vi "Measurement_R2.vi"(0 "I offset":dbl, 1 "PID gains":T1={"proportional gain (Kc)"=1.0, "integral time (Ti, min)"=0.01, "derivative time (Td, min)"=0.0} {"derivative time (Td, min)" format="%.3f"; "integral time (Ti, min)" format="%.3f"; "proportional gain (Kc)" format="%.3f"}, 2 "input cluster":T2) -> (3 "VR frequency":dbl, 4 "VL frequency":dbl, 5 "PLL output":cluster{dbl, dbl, dbl, dbl}, 6 "RMS values":dbl[](array[numeric]), 8 "Total power values":dbl[](array[numeric]))   [LabVIEW 2016]
uses:
  <vilib>/ptbypt/NI_PtbyPt.lvlib
panel:
  out "RMS":fxp<+,55,5>
  in  "output cluster":cluster{"reinitialize? (F)":bool, "dt (s)":dbl}
  out "I RMS":dbl
  out "VR RMS":dbl
  out "VL RMS":dbl
  out "Active Power":dbl
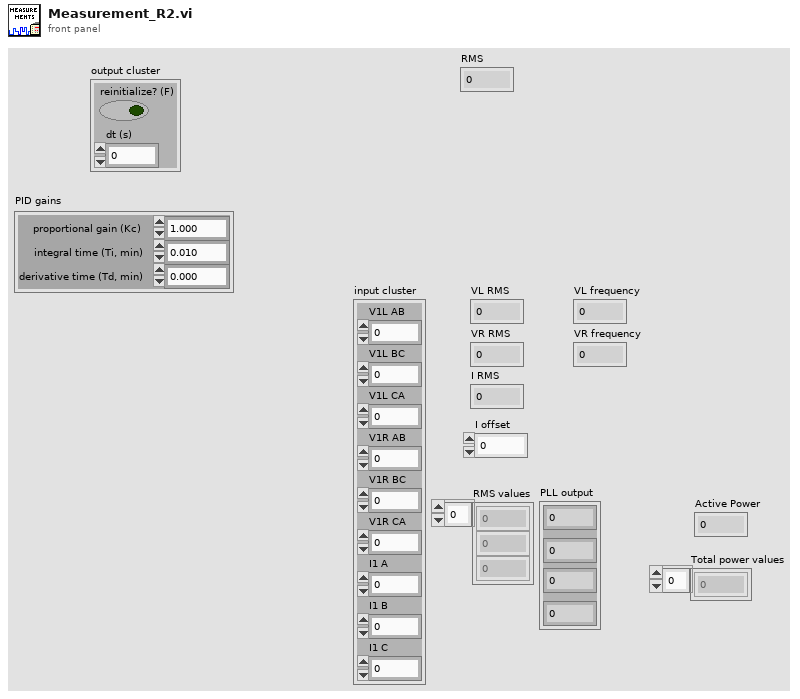
[diagram p1: front panel]
types:
  T1 = cluster{"proportional gain (Kc)":dbl, "integral time (Ti, min)":dbl, "derivative time (Td, min)":dbl}
  T2 = cluster{"V1L AB":fxp<+/-,53,11>, "V1L BC":fxp<+/-,53,11>, "V1L CA":fxp<+/-,53,11>, "V1R AB":fxp<+/-,53,11>, "V1R BC":fxp<+/-,53,11>, "V1R CA":fxp<+/-,53,11>, "I1 A":fxp<+/-,53,11>, "I1 B":fxp<+/-,53,11>, "I1 C":fxp<+/-,53,11>}
  T3 = cluster{fxp<+/-,53,11>, fxp<+/-,53,11>, fxp<+/-,53,11>}
  T4 = cluster{"V1L AB":fxp<+/-,53,11>, "V1L BC":fxp<+/-,53,11>, "V1L CA":fxp<+/-,53,11>}
  T5 = cluster{"V1R AB":fxp<+/-,53,11>, "V1R BC":fxp<+/-,53,11>, "V1R CA":fxp<+/-,53,11>}
  T6 = cluster{"I1 A":fxp<+/-,53,11>, "I1 B":fxp<+/-,53,11>, "I1 C":fxp<+/-,53,11>}
  T7 = cluster{"Frequency":dbl, "Phase":dbl, "Frequency":dbl, "Phase":dbl}
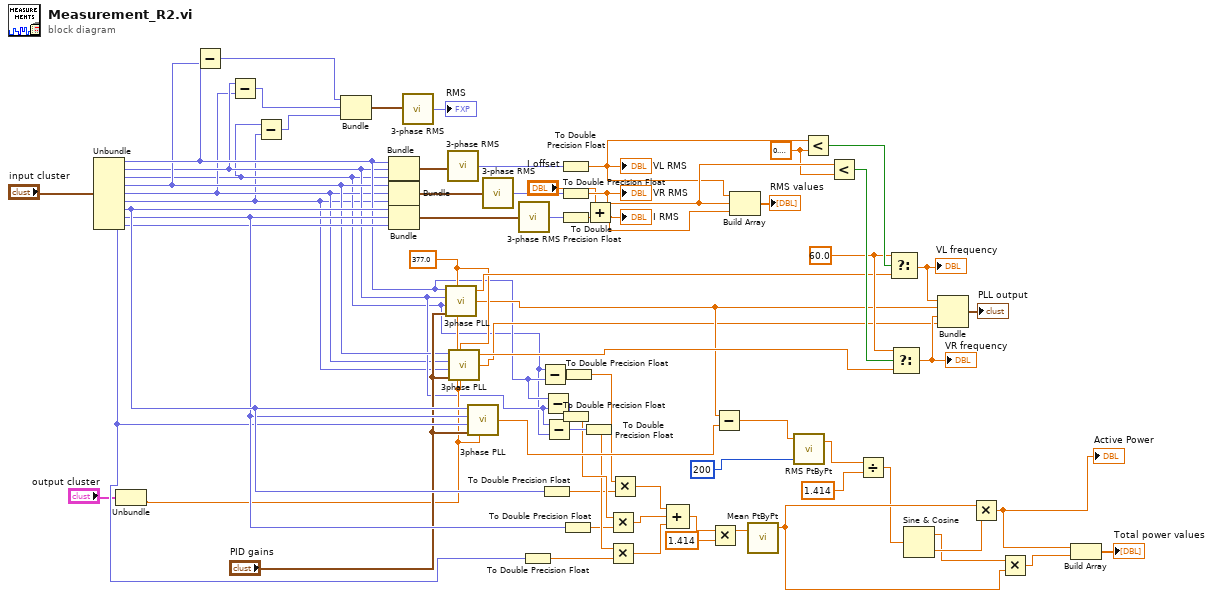
[diagram p0: block diagram]
diagram:
  w50 = 377.0 ("wo")
  w57 = 60.0 ("t")
  w60 = 0.30000001192092896 ("y")
  n1 = Unbundle("input cluster") -> ("V1L AB"=w11:fxp<+/-,53,11>, "V1L BC"=w8:fxp<+/-,53,11>, "V1L CA"=w5:fxp<+/-,53,11>, "V1R AB"=w10:fxp<+/-,53,11>, "V1R BC"=w7:fxp<+/-,53,11>, "V1R CA"=w4:fxp<+/-,53,11>, "I1 A"=w46:fxp<+/-,53,11>, "I1 B"=w45:fxp<+/-,53,11>, "I1 C"=w44:fxp<+/-,53,11>)
  n2 = Unbundle("output cluster") -> ("dt (s)"=w40:dbl)  [unwired: 1 out]
  n3 = Subtract(x=w11, y=w10) -> (x-y=w9:fxp<+/-,53,11>)
  n4 = Subtract(x=w8, y=w7) -> (x-y=w6:fxp<+/-,53,11>)
  n5 = Subtract(x=w5, y=w4) -> (x-y=w3:fxp<+/-,53,11>)
  n6 = Bundle(w9, w6, w3) -> (w2:T3)  [unwired: 1 in]
  n7 = Bundle("V1L AB"=w11, "V1L BC"=w8, "V1L CA"=w5) -> (w68:T4)  [unwired: 1 in]
  n8 = Bundle("V1R AB"=w10, "V1R BC"=w7, "V1R CA"=w4) -> (w67:T5)  [unwired: 1 in]
  n9 = Bundle("I1 A"=w46, "I1 B"=w45, "I1 C"=w44) -> (w66:T6)  [unwired: 1 in]
  n10 = call "3-phase RMS.vi"("Vabc"=w2) -> ("RMS"=→"RMS":fxp<+,55,5>)  [unwired: 4 in]
  n11 = call "3phase PLL.vi"("A"=w11, "wo"=w50, "B"=w8, "C"=w5, "dt (s)"=w40, "PID gains"="PID gains") -> ("Frequency"=w51:dbl, "Phase"=w14:dbl)  [unwired: 1 in]
  n12 = call "3-phase RMS.vi"("Vabc"=w68) -> ("RMS"=w64:fxp<+,55,5>)  [unwired: 4 in]
  n13 = call "3phase PLL.vi"("A"=w10, "wo"=w50, "B"=w7, "C"=w4, "dt (s)"=w40, "PID gains"="PID gains") -> ("Frequency"=w49:dbl, "Phase"=w13:dbl)  [unwired: 1 in]
  n14 = call "3phase PLL.vi"("A"=w46, "B"=w45, "C"=w44, "dt (s)"=w40, "PID gains"="PID gains") -> ("Phase"=w43:dbl)  [unwired: 2 in, 1 out]
  n15 = call "3-phase RMS.vi"("Vabc"=w67) -> ("RMS"=w63:fxp<+,55,5>)  [unwired: 4 in]
  n16 = call "3-phase RMS.vi"("Vabc"=w66) -> ("RMS"=w65:fxp<+,55,5>)  [unwired: 4 in]
  n17 = To Double Precision Float(number=w44) -> (double precision float=w25:dbl)
  n18 = Subtract(x=w5, y=w11) -> (x-y=w39:fxp<+/-,53,11>)
  n19 = To Double Precision Float(number=w46) -> (double precision float=w27:dbl)
  n20 = Subtract(x=w11, y=w8) -> (x-y=w38:fxp<+/-,53,11>)
  n21 = Subtract(x=w8, y=w5) -> (x-y=w37:fxp<+/-,53,11>)
  n22 = To Double Precision Float(number=w64) -> (double precision float=w32:dbl)
  "VL RMS" <- w32
  n23 = To Double Precision Float(number=w63) -> (double precision float=w62:dbl)
  "VR RMS" <- w62
  n24 = To Double Precision Float(number=w65) -> (double precision float=w61:dbl)
  n25 = To Double Precision Float(number=w38) -> (double precision float=w29:dbl)
  n26 = To Double Precision Float(number=w45) -> (double precision float=w26:dbl)
  n27 = To Double Precision Float(number=w39) -> (double precision float=w30:dbl)
  n28 = To Double Precision Float(number=w37) -> (double precision float=w28:dbl)
  n29 = Add(x="I offset", y=w61) -> (x+y=w31:dbl)
  "I RMS" <- w31
  n30 = Multiply(x=w29, y=w26) -> (x*y=w34:dbl)
  n31 = Multiply(x=w28, y=w25) -> (x*y=w33:dbl)
  n32 = Multiply(x=w30, y=w27) -> (x*y=w35:dbl)
  n33 = Compound Arithmetic op=ADD(w35, w34, w33) -> (w24:dbl)
  n34 = Multiply(x=w24, y=1.414) -> (x*y=w18:dbl)
  n35 = Subtract(x=w14, y=w43) -> (x-y=w22:dbl)
  n36 = Build Array(w32, w62, w31) -> (→"RMS values":dbl[])
  n37 = call <vilib>:"Mean PtByPt.vi"("x"=w18) -> ("mean"=w23:dbl)  [unwired: 3 in, 1 out]
  n38 = call <vilib>:"RMS PtByPt.vi"("sample length"=200, "x"=w22) -> ("rms value"=w21:dbl)  [unwired: 2 in, 1 out]
  n39 = Less?(x=w32, y=w60) -> (x < y?=w59:bool)
  n40 = Less?(x=w62, y=w60) -> (x < y?=w58:bool)
  n41 = Divide(x=w21, y=1.414) -> (x/y=w20:dbl)
  n42 = Select(t=w57, s=w59, f=w51) -> (s? t:f=w56:dbl)
  "VL frequency" <- w56
  n43 = Select(t=w57, s=w58, f=w49) -> (s? t:f=w55:dbl)
  "VR frequency" <- w55
  n44 = Sine & Cosine(0:w20) -> (1:w12:dbl, 2:w47:dbl)
  n45 = Bundle("Frequency"=w56, "Phase"=w14, "Frequency"=w55, "Phase"=w13) -> (→"PLL output":T7)  [unwired: 1 in]
  n46 = Multiply(x=w23, y=w47) -> (x*y=w15:dbl)
  "Active Power" <- w15
  n47 = Multiply(x=w12, y=w23) -> (x*y=w36:dbl)
  n48 = Build Array(w15, w36) -> (→"Total power values":dbl[])
